vi "Autonomous Independent.vi"   [LabVIEW 2020]
doc: "This VI is called when autonomous begins, and will automatically be terminated when autonomous ends. You can carry out timed or sensor driven robot movement independently without needing to return to the caller."
uses:
  <vilib>/Rock Robotics/WPI/DriverStation/WPI_DriverStationAllianceInfo.ctl
  Arm/ArmPositionPreset.ctl
  Arm/ArmGamePiecePreset.ctl
  Autonomous/TrajectoryOrientation.ctl
  <vilib>/Rock Robotics/Network Tables/NT Read String.vi
  <vilib>/Rock Robotics/Network Tables/NT Write String.vi
  <vilib>/Rock Robotics/Network Tables/NT Read Number.vi
panel:
  # "Be sure to right-click and choose Data Operations>>Make Current Value default if you want to save the array values with the VI"
types:
  T1 = typedef "WPI_DriverStationAllianceInfo.ctl" = enum16{"Red", "Blue", "Invalid"}
  T2 = typedef "ArmGamePiecePreset.ctl" = enum16{"Cube", "Cone"}
  T3 = typedef "ArmPositionPreset.ctl" = enum16{"Upper", "Lower", "Middle", "Home", "Shelf", "Floor", "HalfFloor", "HalfHome"}
  T4 = typedef "TrajectoryOrientation.ctl" = enum16{"SameOrientation", "RotateToEndOrientation"}
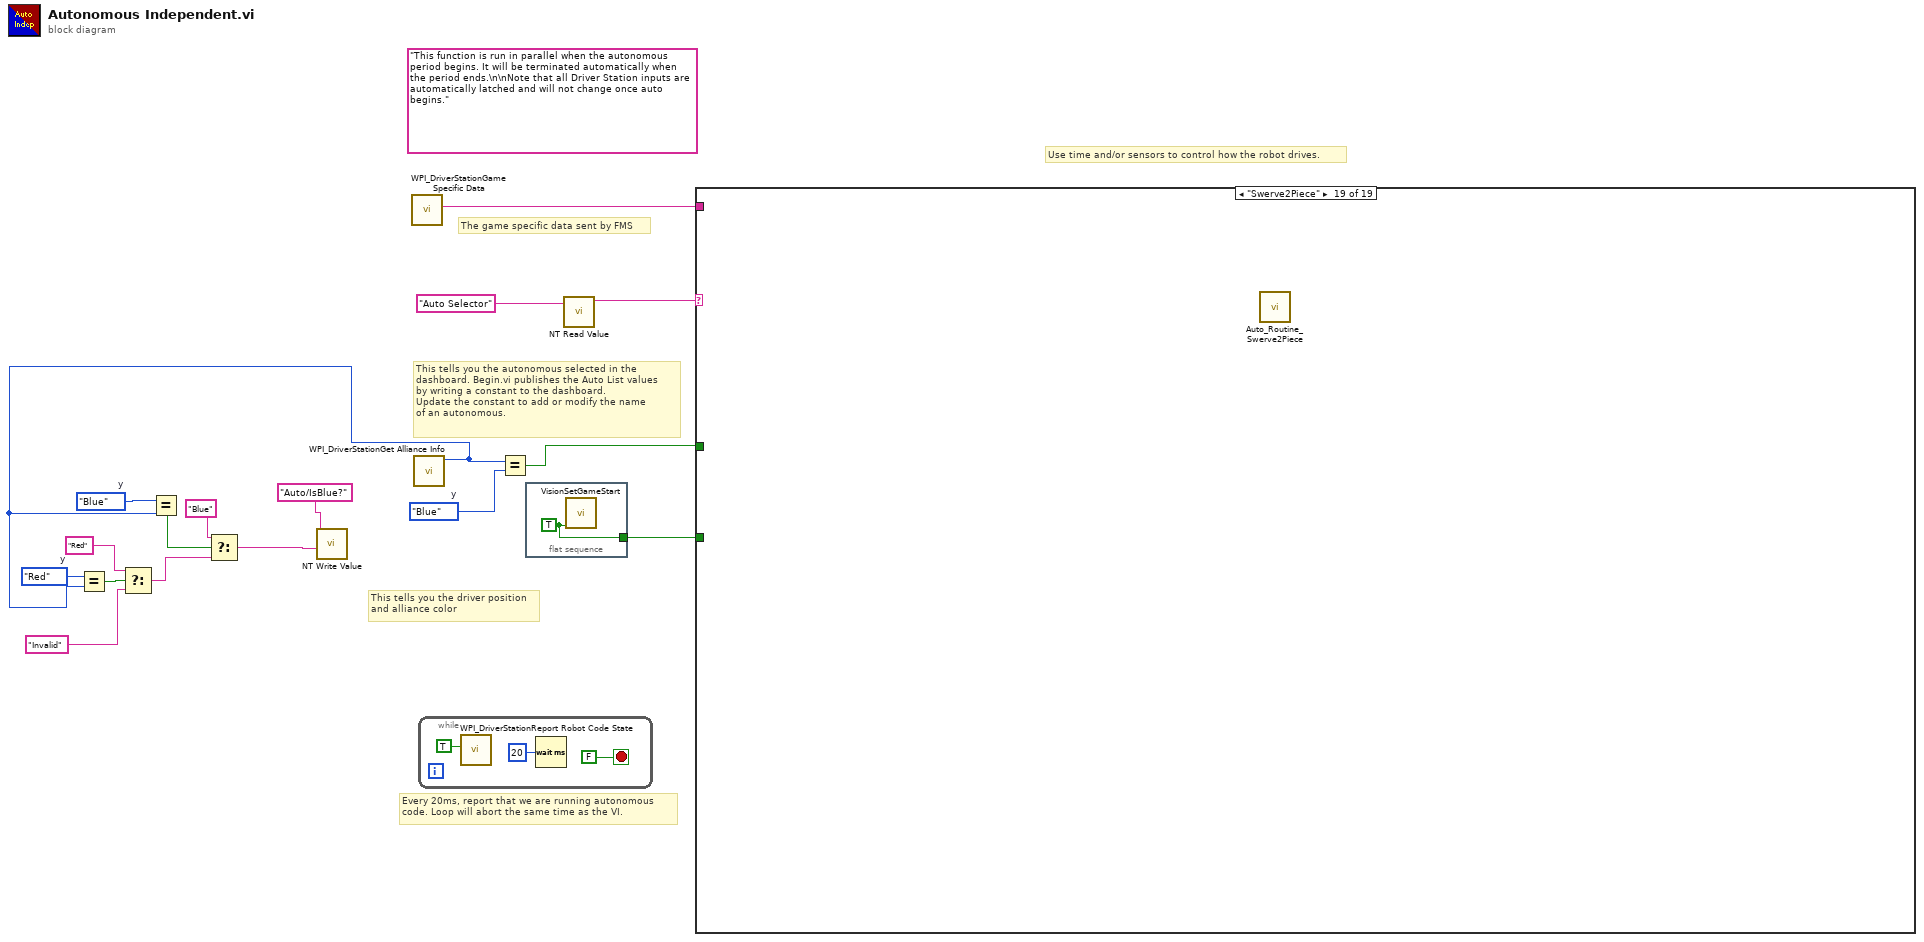
[diagram p0: block diagram]
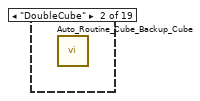
[diagram p3: hidden frame]
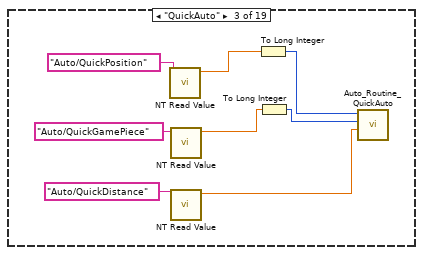
[diagram p4: hidden frame]
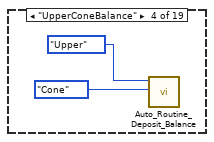
[diagram p5: hidden frame]
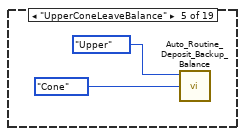
[diagram p6: hidden frame]
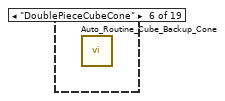
[diagram p7: hidden frame]
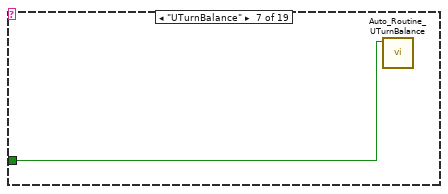
[diagram p8: hidden frame]
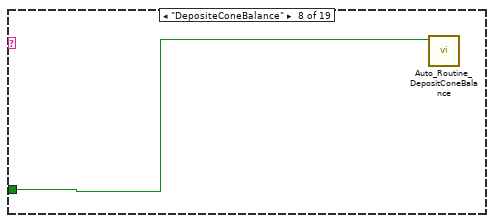
[diagram p9: hidden frame]
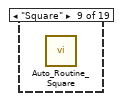
[diagram p10: hidden frame]
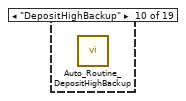
[diagram p11: hidden frame]
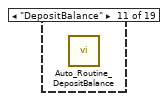
[diagram p12: hidden frame]
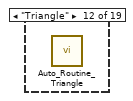
[diagram p13: hidden frame]
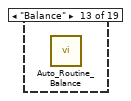
[diagram p14: hidden frame]
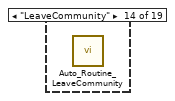
[diagram p15: hidden frame]
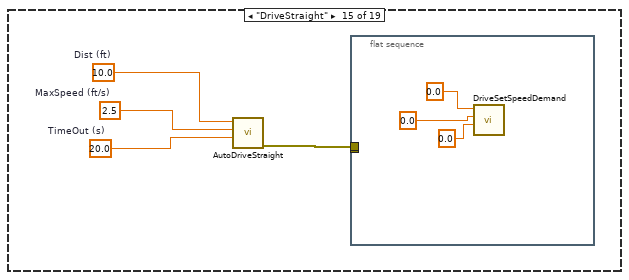
[diagram p16: hidden frame]
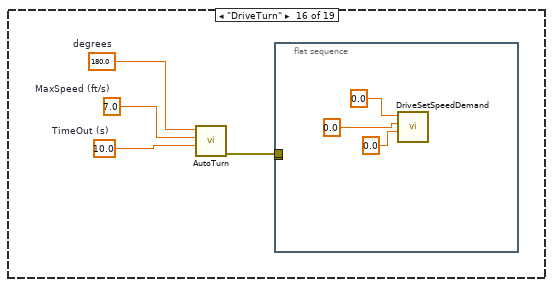
[diagram p17: hidden frame]
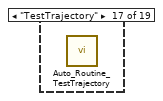
[diagram p18: hidden frame]
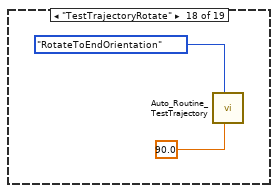
[diagram p19: hidden frame]
diagram:
  w9 = WPI_DriverStationAllianceInfo."Red"  # y
  w11 = WPI_DriverStationAllianceInfo."Blue"  # y
  w14 = WPI_DriverStationAllianceInfo."Blue"  # y
  (unwired) "This function is run in parallel when the autonomous period begins. It will be terminated automatically when the period ends.\n\nNote that all Driver Station inputs are automatically latched and will not change once auto begins."
  # "The game specific data sent by FMS"
  # "This tells you the autonomous selected in the \ndashboard. Begin.vi publishes the Auto List values\nby writing a constant to the dashboard.\nUpdate the constant to add or modify the name\nof an autonomous."
  # "Every 20ms, report that we are running autonomous\ncode. Loop will abort the same time as the VI."
  # "Use time and/or sensors to control how the robot drives."
  # "This tells you the driver position\nand alliance color"
  n1 = call <vilib>:"WPI_DriverStationGame Specific Data.vi"() -> ("Game Specific Data"=w15:string)  [unwired: 11 in]
  n2 = call <vilib>:"WPI_DriverStationGet Alliance Info.vi"() -> ("Alliance"=w3:T1)  [unwired: 11 out]
  n3 = Equal?(x=w9, y=w3) -> (x = y?=w8:bool)
  n4 = Select(t="Red", s=w8, f="Invalid") -> (s? t:f=w12:string)
  n5 = Equal?(x=w11, y=w3) -> (x = y?=w10:bool)
  n6 = Select(t="Blue", s=w10, f=w12) -> (s? t:f=w4:string)
  n7 = call-poly <vilib>:"NT Write Value.vi"("value"=w4, "name"="Auto/IsBlue?") -> ()  [unwired: 9 in, 1 out]
  n8 = while {
    stop <- FALSE stop-if-true
    n9 = call <vilib>:"WPI_DriverStationReport Robot Code State.vi"("Autonomous"=TRUE) -> ()  [unwired: 10 in, 1 out]
    n10 = Wait (ms)(milliseconds to wait=u32 20) -> ()  [unwired: 1 out]
  }
  n11 = Equal?(x=w3, y=w14) -> (x = y?=w2:bool)
  n12 = flat-sequence {
    tunnel: [w21] -> w1
    frame #0 {
      w21 = TRUE ("Game Start")
      n13 = call "VisionSetGameStart.vi"("Game Start"=w21) -> ()  [unwired: 11 in]
    }
  }
  n14 = call-poly <vilib>:"NT Read Value.vi"("name"="Auto Selector" ("Name")) -> ("value"=w16:string)  [unwired: 8 in, 2 out]
  n15 = case shown="\"Swerve2Piece\"" w16 {
    tunnel: w15 -> [_ _ _ _ _ _ _ _ _ _ _ _ _ _ _ _ _ _ _]
    tunnel: w2 -> [_ _ _ _ _ _ w34 w35 _ _ _ _ _ _ _ _ _ _ _]
    tunnel: w1 -> [_ _ _ _ _ _ _ _ _ _ _ _ _ _ _ _ _ _ _]
    frame Default {
      # "You can put your main auto here, or you can right-click on the case and make any\nother frame be the default case."
      # "This is the frame that will execute if no selection is made, or if it is not recognized"
    }
    frame "DoubleCube" {
      n16 = call "Auto_Routine_Cube_Backup_Cube.vi"() -> ()  [unwired: 11 in, 1 out]
    }
    frame "QuickAuto" {
      n17 = call-poly <vilib>:"NT Read Value.vi"("name"="Auto/QuickPosition") -> ("value"=w25:dbl)  [unwired: 8 in, 2 out]
      n18 = call-poly <vilib>:"NT Read Value.vi"("name"="Auto/QuickGamePiece") -> ("value"=w22:dbl)  [unwired: 8 in, 2 out]
      n19 = call-poly <vilib>:"NT Read Value.vi"("name"="Auto/QuickDistance") -> ("value"=w29:dbl)  [unwired: 8 in, 2 out]
      n20 = To Long Integer(number=w25) -> (32bit integer=w24:i32)
      n21 = To Long Integer(number=w22) -> (32bit integer=w23:i32)
      n22 = call "Auto_Routine_QuickAuto.vi"("Distance(Back)"=w29, "Game Piece"=w23, "Position"=w24) -> ()  [unwired: 8 in, 1 out]
    }
    frame "UpperConeBalance" {
      n23 = call "Auto_Routine_Deposit_Balance.vi"("Game Piece"=ArmGamePiecePreset."Cone", "Position"=ArmPositionPreset."Upper") -> ()  [unwired: 9 in, 1 out]
    }
    frame "UpperConeLeaveBalance" {
      n24 = call "Auto_Routine_Deposit_Backup_Balance.vi"("Game Piece"=ArmGamePiecePreset."Cone", "Position"=ArmPositionPreset."Upper") -> ()  [unwired: 9 in, 1 out]
    }
    frame "DoublePieceCubeCone" {
      n25 = call "Auto_Routine_Cube_Backup_Cone.vi"() -> ()  [unwired: 11 in, 1 out]
    }
    frame "UTurnBalance" {
      n26 = call "Auto_Routine_UTurnBalance.vi"("IsBlue?"=w34) -> ()  [unwired: 10 in, 1 out]
    }
    frame "DepositeConeBalance" {
      n27 = call "Auto_Routine_DepositConeBalance.vi"("IsBlue?"=w35) -> ()  [unwired: 10 in, 1 out]
    }
    frame "Square" {
      n28 = call "Auto_Routine_Square.vi"() -> ()  [unwired: 11 in, 1 out]
    }
    frame "DepositHighBackup" {
      n29 = call "Auto_Routine_DepositHighBackup.vi"() -> ()  [unwired: 11 in, 1 out]
    }
    frame "DepositBalance" {
      n30 = call "Auto_Routine_DepositBalance.vi"() -> ()  [unwired: 11 in, 1 out]
    }
    frame "Triangle" {
      n31 = call "Auto_Routine_Triangle.vi"() -> ()  [unwired: 11 in, 1 out]
    }
    frame "Balance" {
      n32 = call "Auto_Routine_Balance.vi"() -> ()  [unwired: 11 in, 1 out]
    }
    frame "LeaveCommunity" {
      n33 = call "Auto_Routine_LeaveCommunity.vi"() -> ()  [unwired: 11 in, 1 out]
    }
    frame "DriveStraight" {
      w37 = 20.0  # TimeOut (s)
      w38 = 2.5  # MaxSpeed (ft/s)
      w39 = 10.0  # Dist (ft)
      n34 = call "AutoDriveStraight.vi"("TimeOut (s)"=w37, "MaxSpeed (ft/s)"=w38, "Dist (ft)"=w39) -> ("error out"=w36:errorcluster)  [unwired: 8 in]
      n35 = flat-sequence {
        tunnel: [w43] -> _
        tunnel: w36 -> [w43]
        frame #0 {
          n36 = call "DriveSetSpeedDemand.vi"("ASpeedDemand (d/s)"=0.0, "YSpeedDemand (ft/s)"=0.0, "XSpeedDemand (ft/s)"=0.0) -> ()  [unwired: 9 in]
        }
      }
    }
    frame "DriveTurn" {
      w45 = 10.0  # TimeOut (s)
      w46 = 7.0  # MaxSpeed (ft/s)
      w47 = 180.0  # degrees
      n37 = call "AutoTurn.vi"("TimeOut (s)"=w45, "MaxSpeed (ft/s)"=w46, "degrees"=w47) -> ("error out"=w44:errorcluster)  [unwired: 8 in]
      n38 = flat-sequence {
        tunnel: [w51] -> _
        tunnel: w44 -> [w51]
        frame #0 {
          n39 = call "DriveSetSpeedDemand.vi"("ASpeedDemand (d/s)"=0.0, "YSpeedDemand (ft/s)"=0.0, "XSpeedDemand (ft/s)"=0.0) -> ()  [unwired: 9 in]
        }
      }
    }
    frame "TestTrajectory" {
      n40 = call "Auto_Routine_TestTrajectory.vi"() -> ()  [unwired: 12 in]
    }
    frame "TestTrajectoryRotate" {
      n41 = call "Auto_Routine_TestTrajectory.vi"("End Orientation"=90.0, "Orientation"=TrajectoryOrientation."RotateToEndOrientation") -> ()  [unwired: 10 in]
    }
    frame "Swerve2Piece" {
      n42 = call "Auto_Routine_Swerve2Piece.vi"() -> ()  [unwired: 11 in, 1 out]
    }
  }
